vi "CPP-13303Spectra.vi"() -> (5 "Plug in titles":string[](array[string]), 7 "Plug in values":string[](array[string]))   [LabVIEW 2018]
uses:
  Globals/Meas_global.vi
panel:
  out "dF":dbl
  out "Ch2BMeanSpec":dbl[](array[numeric])
  out "Ch1CMeanSpec":dbl[](array[numeric])
  in  "Tab Control":enum32{"Graphs", "Numerics"}(tab)
  out "Spectra":T1(graph)
  out "Timetrace":dbl[][](graph)
  in  "Save Button":bool=TRUE
  out "Ch3AMeanSpec":dbl[](array[numeric])
  out "Ch0DMeanSpec":dbl[](array[numeric])
  in  "Band1Start":dbl=3425.0 format="%#_13g"
  in  "Band1Width":dbl=20.0 format="%#_13g"
  # "Please make sure to set a valid path, otherwise spectra will not be saved, silently"
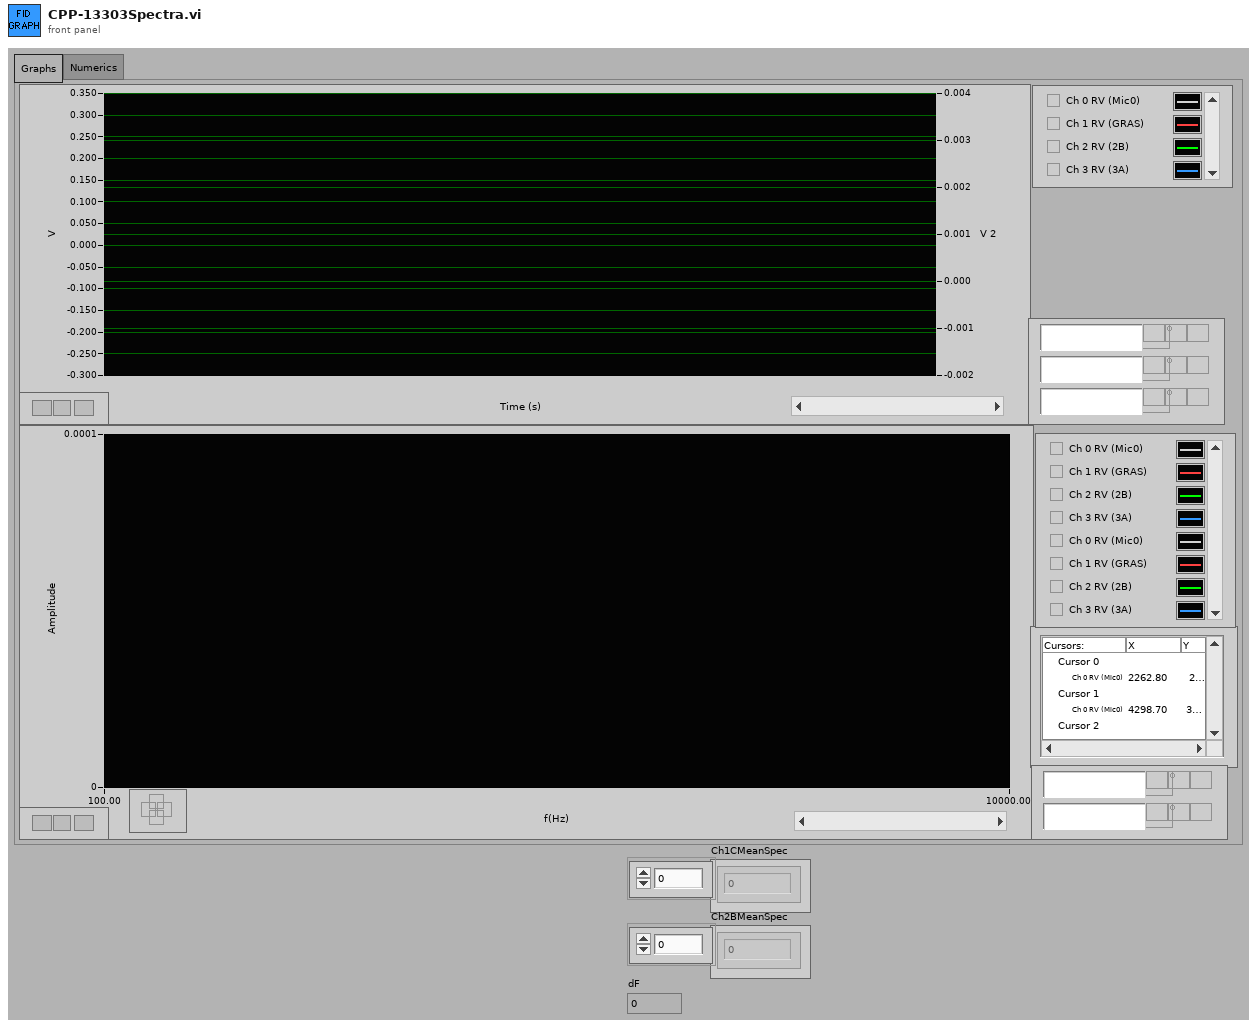
[diagram p1: front panel]
types:
  T1 = cluster{"dF":dbl, "dF":dbl, "Spectrum output array":dbl[]}[]
  T2 = typedef "Analysis_info_cluster.ctl" = cluster{"Colour":u32, "Inst type":T3, "Inst name":string, "Symbol":string, "Code name":string, "Extra Info":string, "Inst Array":T4, "Extra Titles":string[], "Extra Values":string[], "U":dbl, "u^2":dbl, "u^3":dbl, "u^4":dbl, "Skew_u":dbl, "Kurt_u":dbl, "Sd Error in Mean":dbl, "% u'/U":dbl, "X":dbl, "Y":dbl, "Z":dbl, "Timescale integral Estimate":dbl, "Sd Error in Variance":dbl, "Calib File":path, "Calib Constants":dbl[], "Output Position":bool, "Stats":enum16{"None", "Basic", "Full"}, "Av Sampling Rate":dbl, "Av No of Samples":dbl, "Total Meas Time (s)":dbl, "ADAM Ch Name":string, "Max value":dbl, "Min value":dbl, "Req Sample Rate Hz":dbl, "Sync Delay Time (s)":dbl, "Ch No":i16, "Device":string, "Use Latest Calib":bool, "Port":string, "Metadata Ch Names":string[], "Metadata Ch Values":string[]}
  T3 = typedef "Inst_type.ctl" = enum16{"Propeller anemometer", "Raw voltage", "Pressure Transducer", "Pitot-static tube", "Preston tube", "Hot wire", "Cross wire 1", "Cross wire 2", "Generic Linear", "Generic Polynomial", "Generic BackPoly", "Fast FID", "Thermocouple", "Cold wire", "Pulsed Wire", "LDA Vel", "LDA Tran time", "LDA Arr time", "Microphone"}
  T4 = typedef "Instrument_Array.ctl" = enum16{"PWA", "LDA", "Analogue"}
  T5 = enum16{"Save no data", "Save data in new files", "Save data in existing files"}
  T6 = typedef "Time_Trace_Cluster.ctl" = cluster{"Weighting":dbl[], "Time (s)":dbl[], "Voltage":dbl[], "Eng Values":dbl[]}
  T7 = cluster{"dF":dbl, "dF":dbl, "SingleBlockSpectrum":dbl[]}
  T8 = cluster{"dF":dbl, "dF":dbl, "SingleBlockSpectrum":dbl[]}[]
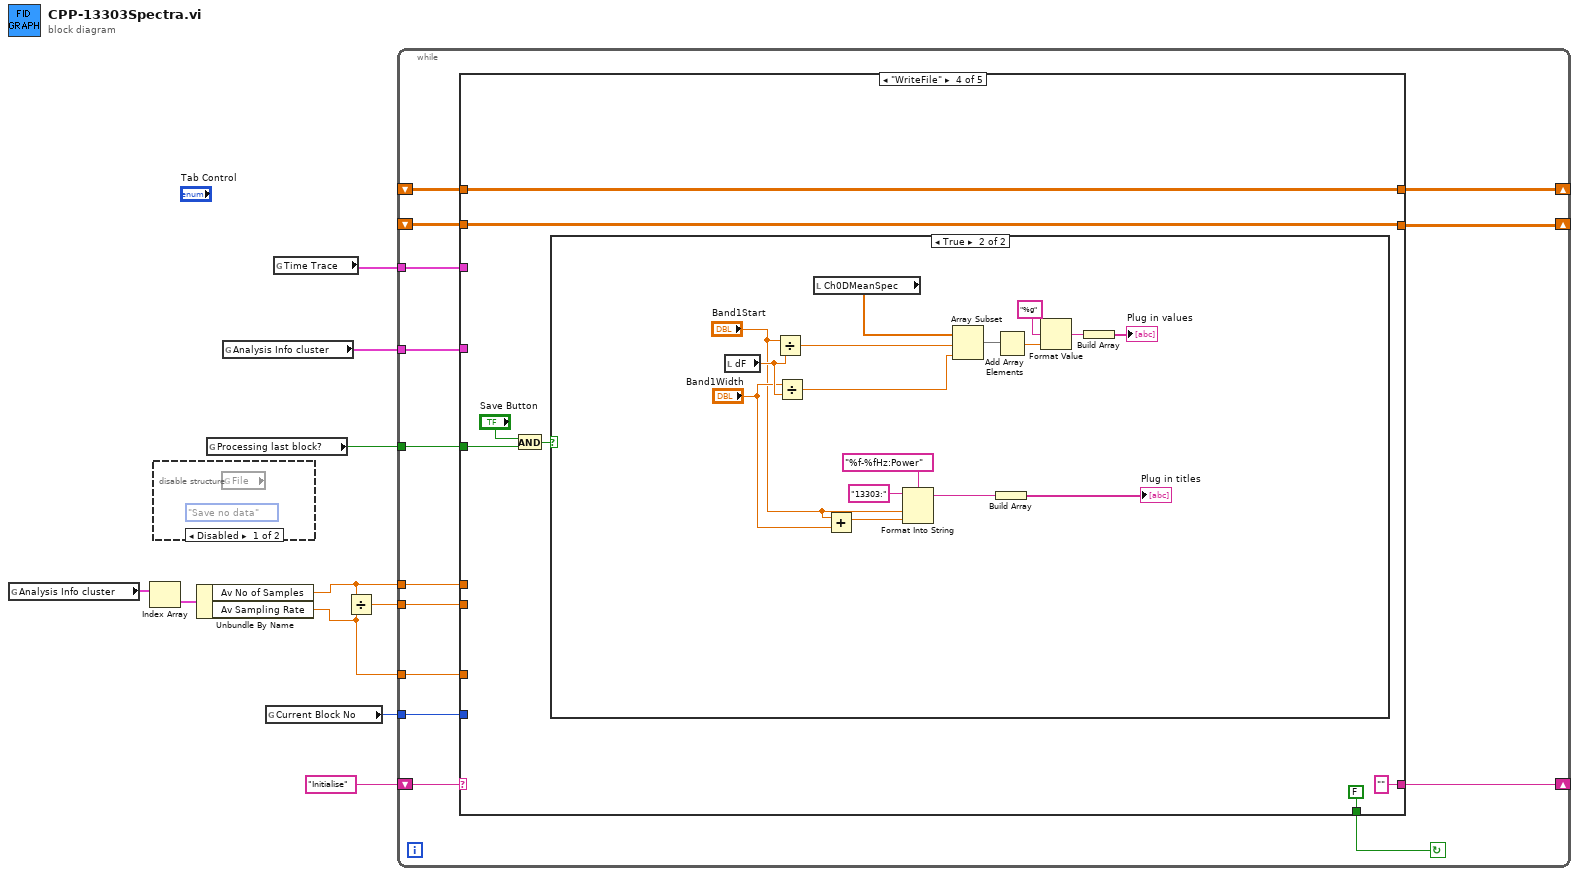
[diagram p0: block diagram]
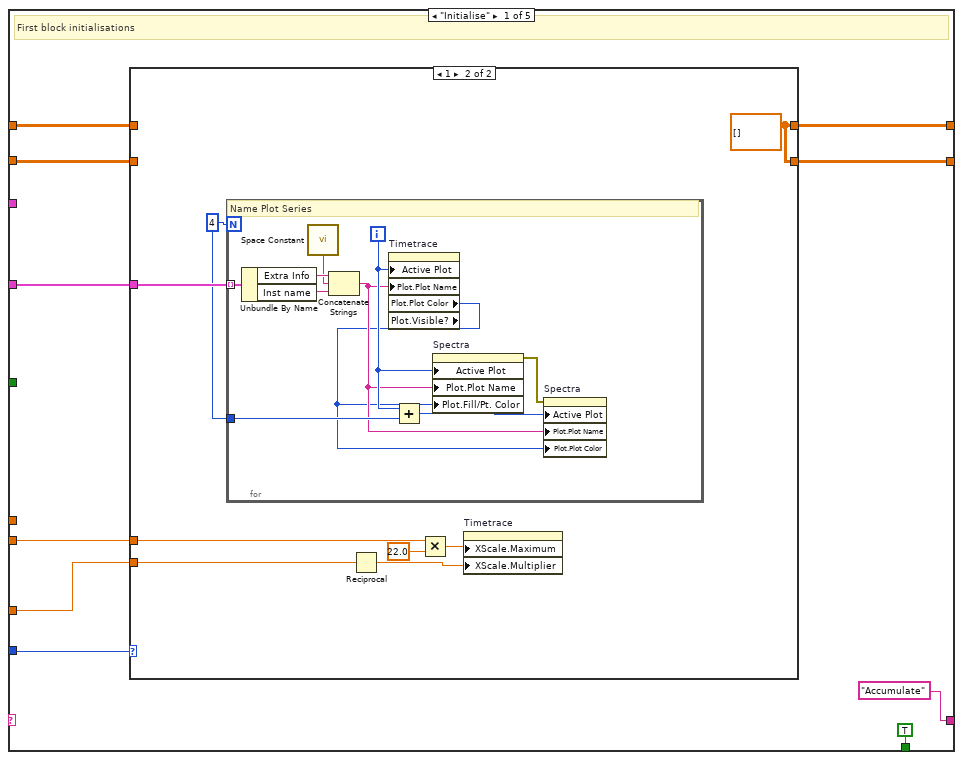
[diagram p3: hidden frame]
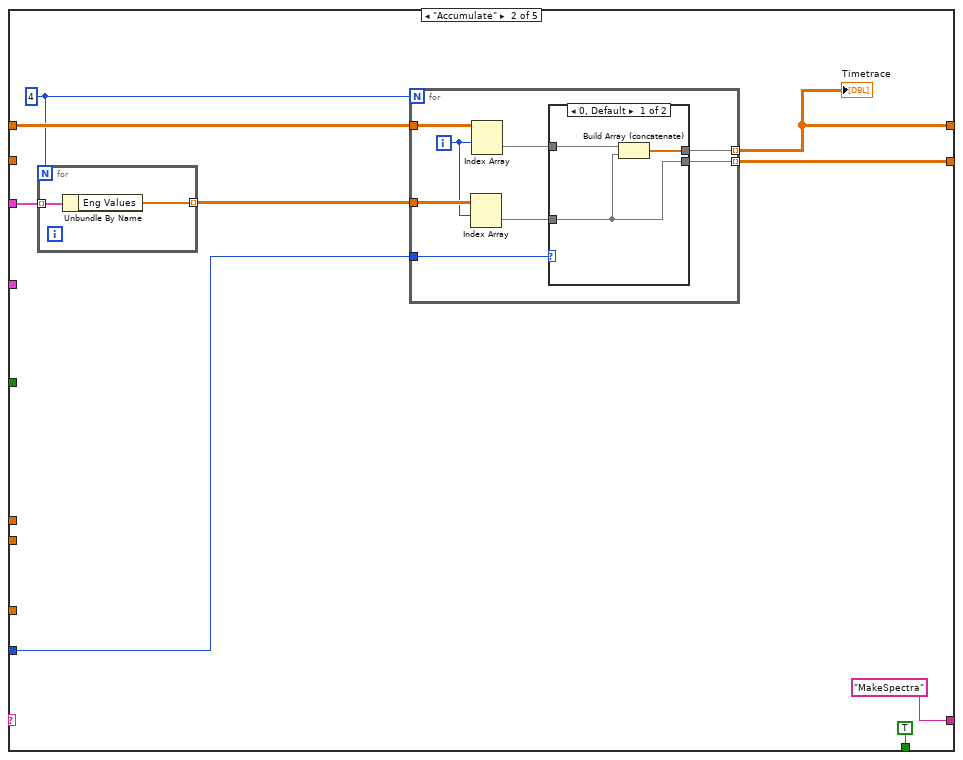
[diagram p5: hidden frame]
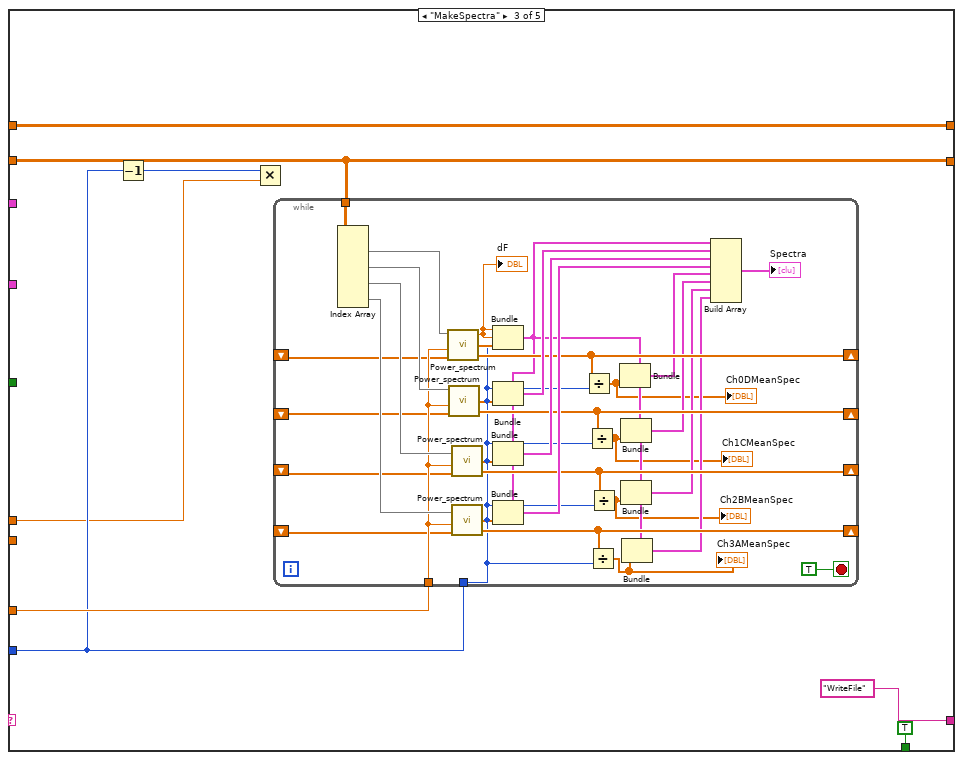
[diagram p7: hidden frame]
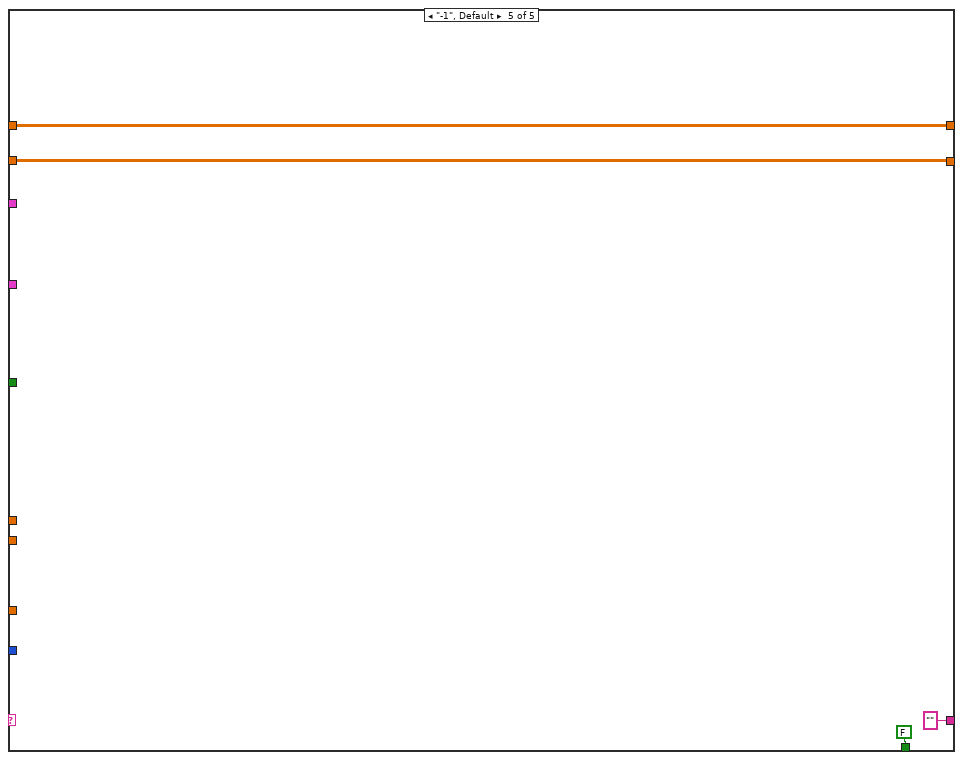
[diagram p9: hidden frame]
diagram:
  n1 = global read "Meas_global.vi" "Analysis Info cluster"() -> (w4:T2[])
  n2 = Index Array(array=w4) -> (element=w3:T2)  [unwired: 1 in]
  n3 = disable-structure shown="Disabled" {
    frame Disabled {
      (unwired) T5."Save no data" ("File")
      n4 = global read "Meas_global.vi" "File"() -> ()  [unwired: 1 out]
    }
    frame Enabled {
    }
  }
  n5 = Unbundle By Name(w3) -> ("Av No of Samples"=w2:dbl, "Av Sampling Rate"=w1:dbl)
  n6 = global read "Meas_global.vi" "Processing last block?"() -> (w5:bool)
  n7 = global read "Meas_global.vi" "Analysis Info cluster"() -> (w7:T2[])
  n8 = global read "Meas_global.vi" "Current Block No"() -> (w9:i32)
  n9 = global read "Meas_global.vi" "Time Trace"() -> (w10:T6[])
  n10 = Divide(x=w2, y=w1) -> (x/y=w8:dbl)
  n11 = while {
    shift-left: "Initialise" -> [w16]
    shift-right: [w22] -> _
    tunnel: w10 -> [w23]
    tunnel: w9 -> [w21]
    tunnel: w8 -> [w20]
    shift-right: [w18] -> _
    shift-left: _ -> [w19]
    tunnel: w7 -> [w17]
    tunnel: w5 -> [w15]
    tunnel: w1 -> [w14]
    tunnel: w2 -> [w13]
    shift-right: [w12] -> _
    shift-left: _ -> [w11]
    stop <- w24 continue-if-true
    n12 = case shown="\"WriteFile\"" w16 {
      tunnel: [TRUE TRUE TRUE FALSE FALSE] -> w24
      tunnel: w23 -> [_ w63 _ _ _]
      tunnel: ["Accumulate" "MakeSpectra" "WriteFile" "" ""] -> w22
      tunnel: w21 -> [w29 w59 w81 _ _]
      tunnel: w20 -> [w33 _ _ _ _]
      tunnel: w17 -> [w31 _ _ _ _]
      tunnel: [w32 w57 w83 w126 w145] -> w18
      tunnel: w19 -> [w28 w58 w83 w126 w145]
      tunnel: w15 -> [_ _ _ w122 _]
      tunnel: w14 -> [w27 _ w82 _ _]
      tunnel: w13 -> [_ _ w80 _ _]
      tunnel: [w26 w55 w78 w125 w143] -> w12
      tunnel: w11 -> [w25 _ w78 w125 w143]
      frame "Initialise" {
        # "First block initialisations"
        n13 = case shown="1" w29 {
          tunnel: w33 -> [_ w43]
          tunnel: [w36 w37] -> w32
          tunnel: w31 -> [_ w42]
          tunnel: w28 -> [w36 _]
          tunnel: w27 -> [_ w39]
          tunnel: [w35 w37] -> w26
          tunnel: w25 -> [w35 _]
          frame 0, Default {
          }
          frame 1 {
            w37 = dbl[][] [] ("Eng Values")
            w38 = 4
            n14 = for {
              N: w38 -> [_]
              tunnel: w42 -> [w52] mode=indexing
              tunnel: w38 -> [w49]
              i -> [w50]
              # "Name Plot Series"
              n15 = Unbundle By Name(w52) -> ("Extra Info"=w54:string, "Inst name"=w51:string)
              n16 = call <vilib>:"Space Constant.vi"() -> ("String"=w53:string)
              n17 = Concatenate Strings(w54, w53, w51) -> (w47:string)
              n18 = property on="Timetrace" class="WFGraph (strict)" props=["Active Plot", "Plot", "Plot Name", "Plot", "Plot Color", "Plot", "Visible?"]("Active Plot"=w50, "Plot.Plot Name"=w47) -> ("Plot.Plot Color"=w45:u32)  [unwired: 2 in, 3 out]
              n19 = Add(x=w50, y=w49) -> (x+y=w46:i32)
              n20 = property on="Spectra" class="WFGraph (strict)"("Active Plot"=w50, "Plot.Plot Name"=w47, "Plot.Fill/Pt. Color"=w45) -> (error out=w48:errorcluster)  [unwired: 2 in, 1 out]
              n21 = property on="Spectra" class="WFGraph (strict)"(error in=w48, "Active Plot"=w46, "Plot.Plot Name"=w47, "Plot.Plot Color"=w45) -> ()  [unwired: 1 in, 2 out]
            }
            n22 = Reciprocal(x=w39) -> (1/x=w40:dbl)
            n23 = Multiply(x=w43, y=22.0) -> (x*y=w44:dbl)
            n24 = property on="Timetrace" class="WFGraph (strict)"("XScale.Maximum"=w44, "XScale.Multiplier"=w40) -> ()  [unwired: 2 in, 2 out]
          }
        }
      }
      frame "Accumulate" {
        w56 = 4
        n25 = for {
          N: w56 -> [_]
          tunnel: w63 -> [w77] mode=indexing
          tunnel: [w76] -> w60 mode=indexing
          n26 = Unbundle By Name(w77) -> ("Eng Values"=w76:dbl[])
        }
        n27 = for {
          N: w56 -> [_]
          tunnel: w60 -> [w71]
          tunnel: [w70] -> w57 mode=indexing
          tunnel: w59 -> [w68]
          tunnel: w58 -> [w66]
          tunnel: [w64] -> w55 mode=indexing
          i -> [w65]
          n28 = Index Array(array=w71, index (row)=w65) -> (element=w67:dbl[])  [unwired: 1 in]
          n29 = Index Array(array=w66, index (row)=w65) -> (element=w69:dbl[])  [unwired: 1 in]
          n30 = case shown="0, Default" w68 {
            tunnel: w69 -> [w74 _]
            tunnel: w67 -> [w72 w75]
            tunnel: [w73 w75] -> w70
            tunnel: [w72 w75] -> w64
            frame 0, Default {
              n31 = Build Array (concatenate)(w74, w72) -> (w73:dbl[])
            }
            frame 1 {
            }
          }
        }
        "Timetrace" <- w57
      }
      frame "MakeSpectra" {
        n32 = Decrement(x=w81) -> (x-1=w79:i32)
        n33 = Multiply(x=w79, y=w80) -> ()  [unwired: 1 out]
        n34 = while {
          tunnel: w78 -> [w119]
          tunnel: w82 -> [w111]
          tunnel: w81 -> [w96]
          shift-right: [w101] -> _
          shift-left: _ -> [w106]
          shift-right: [w100] -> _
          shift-left: _ -> [w105]
          shift-right: [w99] -> _
          shift-left: _ -> [w104]
          shift-right: [w98] -> _
          shift-left: _ -> [w103]
          stop <- TRUE stop-if-true
          n35 = Index Array(array=w119) -> (element #1=w118:dbl[], element #2=w117:dbl[], element #3=w116:dbl[], element #4=w112:dbl[])  [unwired: 8 in]
          n36 = call "Power_spectrum.vi"("U"=w118, "Sampling frequency"=w111, "Spectrum input array"=w106, "Block No"=w96) -> ("dF"=w90:dbl, "SingleBlockSpectrum"=w109:dbl[], "Spectrum Accumulator array"=w101:dbl[])  [unwired: 1 in]
          "dF" <- w90
          n37 = call "Power_spectrum.vi"("U"=w117, "Sampling frequency"=w111, "Spectrum input array"=w105, "Block No"=w96) -> ("SingleBlockSpectrum"=w102:dbl[], "Spectrum Accumulator array"=w100:dbl[])  [unwired: 1 in, 1 out]
          n38 = call "Power_spectrum.vi"("U"=w116, "Sampling frequency"=w111, "Spectrum input array"=w104, "Block No"=w96) -> ("SingleBlockSpectrum"=w108:dbl[], "Spectrum Accumulator array"=w99:dbl[])  [unwired: 1 in, 1 out]
          n39 = call "Power_spectrum.vi"("U"=w112, "Sampling frequency"=w111, "Spectrum input array"=w103, "Block No"=w96) -> ("SingleBlockSpectrum"=w107:dbl[], "Spectrum Accumulator array"=w98:dbl[])  [unwired: 1 in, 1 out]
          n40 = Bundle("dF"=w90, "dF"=w90, "SingleBlockSpectrum"=w109) -> (w89:T7)  [unwired: 1 out]
          n41 = Bundle(cluster=w89, "SingleBlockSpectrum"=w102) -> (w115:T7)  [unwired: 2 out]
          n42 = Bundle(cluster=w89, "SingleBlockSpectrum"=w108) -> (w114:T7)  [unwired: 2 out]
          n43 = Bundle(cluster=w89, "SingleBlockSpectrum"=w107) -> (w110:T7)  [unwired: 2 out]
          n44 = Divide(x=w101, y=w96) -> (x/y=w88:dbl[])
          "Ch0DMeanSpec" <- w88
          n45 = Divide(x=w100, y=w96) -> (x/y=w87:dbl[])
          "Ch1CMeanSpec" <- w87
          n46 = Divide(x=w98, y=w96) -> (x/y=w97:dbl[])
          "Ch3AMeanSpec" <- w97
          n47 = Divide(x=w99, y=w96) -> (x/y=w86:dbl[])
          "Ch2BMeanSpec" <- w86
          n48 = Bundle(cluster=w89, "SingleBlockSpectrum"=w88) -> (w95:T7)  [unwired: 2 out]
          n49 = Bundle(cluster=w89, "SingleBlockSpectrum"=w87) -> (w94:T7)  [unwired: 2 out]
          n50 = Bundle(cluster=w89, "SingleBlockSpectrum"=w86) -> (w93:T7)  [unwired: 2 out]
          n51 = Bundle(cluster=w89, "SingleBlockSpectrum"=w97) -> (w92:T7)  [unwired: 2 out]
          n52 = Build Array(w89, w115, w114, w110, w95, w94, w93, w92) -> (→"Spectra":T8)
        }
      }
      frame "WriteFile" {
        n53 = And(x="Save Button", y=w122) -> (x .and. y?=w121:bool)
        n54 = case shown="True" w121 {
          frame False {
          }
          frame True {
            n55 = local read "dF"() -> (w136:dbl)
            n56 = Divide(x="Band1Start", y=w136) -> (x/y=w134:dbl)
            n57 = Divide(x="Band1Width", y=w136) -> (x/y=w135:dbl)
            n58 = local read "Ch0DMeanSpec"() -> (w142:dbl[])
            n59 = Add(x="Band1Start", y="Band1Width") -> (x+y=w131:dbl)
            n60 = Format Into String(format string="%f-%fHz:Power", initial string="13303:", "Band1Start", w131) -> (resulting string=w129:string)  [unwired: 1 in, 1 out]
            n61 = Array Subset(array=w142, index=w134, length=w135) -> (w141:dbl[])
            n62 = Build Array(w129) -> (→"Plug in titles":string[])
            n63 = Add Array Elements(numeric array=w141) -> (sum=w140:dbl)
            n64 = Format Value(format string="%g", value (0)=w140) -> (output string=w139:string)  [unwired: 1 in]
            n65 = Build Array(w139) -> (→"Plug in values":string[])
          }
        }
      }
      frame "-1", Default {
      }
    }
  }
